vi "set speed.vi"(8 "error in (no error)":errorcluster, 10 "Speed [rpm]":dbl, 11 "CL57RS in":refnum<class "CL57RS.lvclass">) -> (0 "error out":errorcluster, 3 "CL57RS out":refnum<class "CL57RS.lvclass">)   [LabVIEW 2025, in "Motor.lvlib" / "CL57RS.lvclass"]
uses:
  CL57RS.lvclass
  CL57RS.lvclass/CL57RS.ctl
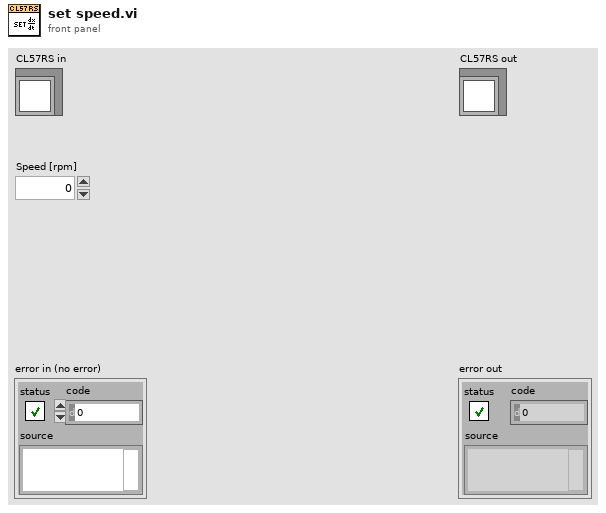
[diagram p1: front panel]
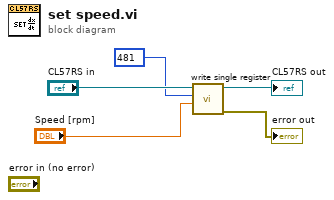
[diagram p0: block diagram]
diagram:
  n1 = call "write single register.vi"("register to write"="Speed [rpm]", "address"=u16 481, "CL57RS in"="CL57RS in") -> ("error out"=→"error out":errorcluster, "CL57RS out"=→"CL57RS out":refnum<class "CL57RS.lvclass">)  [unwired: 7 in]
